vi "HEX2PWL.vi"(11 "data":i32[](array[numeric])) -> (3 "PWL DATA":T1(array[cluster]))   [LabVIEW 2020]
panel:
  out "AMP":dbl
  out "Ramp":u16(ring)=2 items=["Step"=0, "Ramp (Lin.)"=2, "Ramp (Exp.)"=3]
  out "Shape":u16(ring) items=["Sine", "Square"]
  out "freqeuncy":u64
  out "cycle":dbl
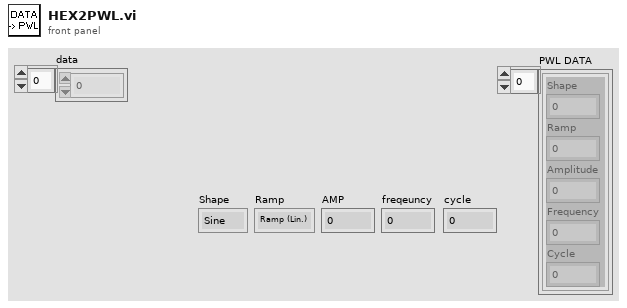
[diagram p1: front panel]
types:
  T1 = cluster{"Shape":u16, "Ramp":u16, "Amplitude":dbl, "Frequency":dbl, "Cycle":dbl}[]
  T2 = cluster{"Shape":u16, "Ramp":u16, "Amplitude":dbl, "Frequency":dbl, "Cycle":dbl}
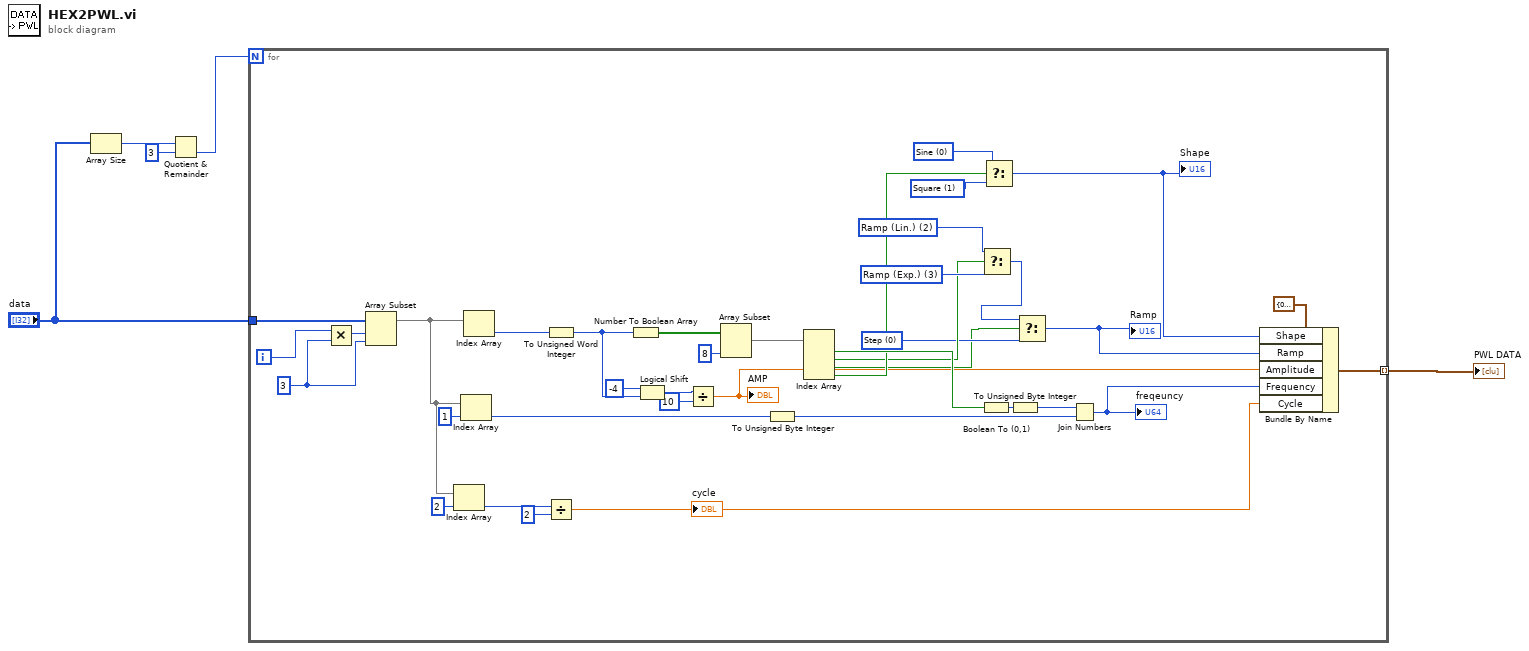
[diagram p0: block diagram]
diagram:
  n1 = Array Size(array="data") -> (size(s)=w3:i32)
  n2 = Quotient & Remainder(x=w3, y=3) -> (floor(x/y)=w1:i32)  [unwired: 1 out]
  n3 = for {
    N: w1 -> [_]
    tunnel: "data" -> [w19]
    tunnel: [w12] -> w5 mode=indexing
    i -> [w10]
    w9 = 3 ("길이")
    w26 = u16 0 items=["Step"=0, "Ramp (Lin.)"=2, "Ramp (Exp.)"=3] ("Ramp")
    w28 = u16 3 items=["Step"=0, "Ramp (Lin.)"=2, "Ramp (Exp.)"=3] ("Ramp")
    w29 = u16 2 items=["Step"=0, "Ramp (Lin.)"=2, "Ramp (Exp.)"=3] ("Ramp")
    w30 = u16 0 items=["Sine", "Square"] ("Shape")
    w32 = u16 1 items=["Sine", "Square"] ("Shape")
    n4 = Multiply(x=w10, y=w9) -> (x*y=w8:i32)
    n5 = Array Subset(array=w19, index=w8, length=w9) -> (w11:i32[])
    n6 = Index Array(array=w11, index=2 ("인덱스")) -> (element=w43:i32)
    n7 = Index Array(array=w11, index=1 ("인덱스")) -> (element=w39:i32)
    n8 = Index Array(array=w11) -> (element=w36:i32)  [unwired: 1 in]
    n9 = To Unsigned Word Integer(number=w36) -> (unsigned 16bit integer=w24:u16)
    n10 = Divide(x=w43, y=2) -> (x/y=w17:dbl)
    "cycle" <- w17
    n11 = Number To Boolean Array(number=w24) -> (Boolean array=w38:bool[])
    n12 = Logical Shift(y=i16 -4, x=w24) -> (x << y=w22:u16)
    n13 = Divide(x=w22, y=u16 10) -> (x/y=w16:dbl)
    "AMP" <- w16
    n14 = Array Subset(array=w38, length=8 ("길이")) -> (w35:bool[])  [unwired: 1 in]
    n15 = To Unsigned Byte Integer(number=w39) -> (unsigned 8bit integer=w6:u8)
    n16 = Index Array(array=w35) -> (element #1=w34:bool, element #2=w27:bool, element #3=w25:bool, element #4=w31:bool)  [unwired: 4 in]
    n17 = Boolean To (0,1)(Boolean=w34) -> (0, 1=w33:i16)
    n18 = Select(t=w29, s=w27, f=w28) -> (s? t:f=w20:u16)
    n19 = Select(t=w30, s=w31, f=w32) -> (s? t:f=w13:u16)
    "Shape" <- w13
    n20 = To Unsigned Byte Integer(number=w33) -> (unsigned 8bit integer=w7:u8)
    n21 = Select(t=w20, s=w25, f=w26) -> (s? t:f=w14:u16)
    "Ramp" <- w14
    n22 = Join Numbers(hi=w7, lo=w6) -> ((hi.lo)=w15:u16)
    "freqeuncy" <- w15
    n23 = Bundle By Name(cluster=T2 {"Shape"=0, "Ramp"=0, "Amplitude"=0.0, "Frequency"=40.0, "Cycle"=1.0} ("Text_File_PWL_DW7802"), "Shape"=w13, "Ramp"=w14, "Amplitude"=w16, "Frequency"=w15, "Cycle"=w17) -> (w12:T2)
  }
  "PWL DATA" <- w5
